vi "Verify Radar Plot.vi"(1 "[user-specified font]":T1={"Font Name:"="Current Font", "Size"=36, "Strikeout?"=FALSE, "Italic?"=FALSE, "Underline?"=FALSE, "Outline?"=TRUE, "Shadow?"=TRUE, "Bold?"=TRUE}, 2 "desired font(Application)":T2(ring), 3 "Text To Draw":string) -> (0 "Radar Plot":picture)   [LabVIEW 2011]
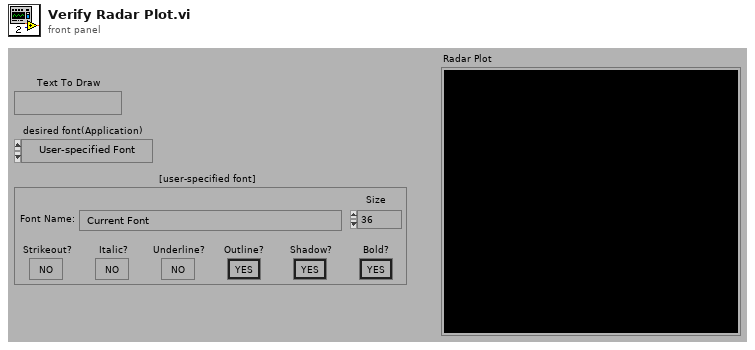
[diagram p1: front panel]
types:
  T1 = cluster{"Font Name:":string, "Size":i16, "Strikeout?":bool, "Italic?":bool, "Underline?":bool, "Outline?":bool, "Shadow?":bool, "Bold?":bool}
  T2 = enum16{"User-specified Font", "Application Font", "System Font", "Dialog Font"}
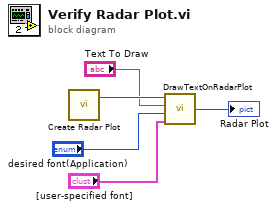
[diagram p0: block diagram]
diagram:
  n1 = call "Create Radar Plot.vi"() -> ("Radar Plot"=w5:picture)  [unwired: 3 out]
  n2 = call "DrawTextOnRadarPlot.vi"("[user-specified font]"="[user-specified font]", "desired font(Application)"="desired font(Application)", "Text To Draw"="Text To Draw", "Radar Plot In"=w5) -> ("Radar Plot Out"=→"Radar Plot":picture)
